vi "dfd_Interpret All Quantizers.vi"(11 "DFD_QSettings":T6[](array[typedef]) {"source" items=["Coef a/k"=0, "Coef b/v"=7, "Input"=1, "Output"=2, "Multiplicand"=3, "Product"=4, "Sum"=5, "Delay"=6, "Gain"=8]}) -> (3 "Fxp_QSettings":T1 {"source" items=["Coef a/k"=0, "Coef b/v"=7, "Input"=1, "Output"=2, "Multiplicand"=3, "Product"=4, "Sum"=5, "Delay"=6, "Gain"=8]})   [LabVIEW 2017, in "NI_DigFilterLicensed.lvlib"]
uses:
  <vilib>/addons/Digital Filter Design/NI_DigFilterLicensed.lvlib
  <vilib>/addons/Digital Filter Design/_Objects.llb/dfd_Internal Quantization Settings.ctl
  <vilib>/addons/Digital Filter Design/_Objects.llb/dfd_Internal Quantization Srcs.ctl
  <vilib>/addons/Digital Filter Design/SCLCodeGen.llb/Typedefs/dfd_SCL_Quantizers.ctl
  <vilib>/fxp/LVFixedPointRepBitsTypeDef.ctl
  <vilib>/fxp/LVFixedPointQuantizationPolicyTypeDef.ctl
  <vilib>/fxp/LVFixedPointOverflowPolicyTypeDef.ctl
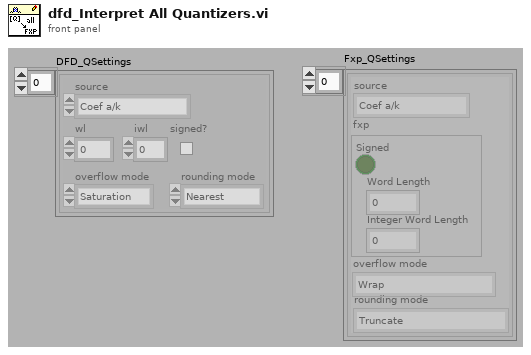
[diagram p1: front panel]
types:
  T1 = typedef "dfd_SCL_Quantizers.ctl" = cluster{"fxp":T2, "rounding mode":T3, "overflow mode":T4, "source":T5}[]
  T2 = typedef "LVFixedPointRepBitsTypeDef.ctl" = cluster{"Signed":bool, "Word Length":u32, "Integer Word Length":i32}
  T3 = typedef "LVFixedPointQuantizationPolicyTypeDef.ctl" = enum32{"Truncate", "Round-Half-Up (Asymmetric)", "Round-Half-Even"}
  T4 = typedef "LVFixedPointOverflowPolicyTypeDef.ctl" = enum32{"Wrap", "Saturate"}
  T5 = typedef "NI_DigFilterLicensed.lvlib/dfd_Internal Quantization Srcs.ctl" = u16
  T6 = typedef "NI_DigFilterLicensed.lvlib/dfd_Internal Quantization Settings.ctl" = cluster{"source":T5, "wl":i16, "iwl":i16, "overflow mode":enum16{"Saturation", "Wrap"}, "rounding mode":enum16{"Nearest", "Truncation"}, "signed?":bool}
  T7 = cluster{"fxp representation":T2, "rounding mode":T3, "overflow mode":T4, "source":T5}
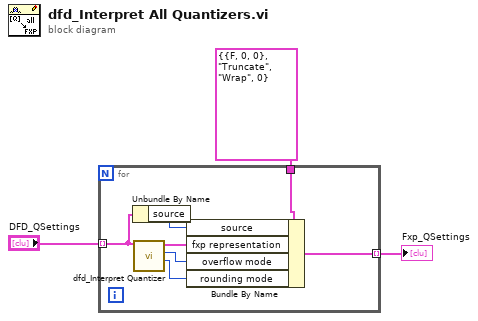
[diagram p0: block diagram]
diagram:
  n1 = for {
    tunnel: "DFD_QSettings" -> [w9] mode=indexing
    tunnel: T7 {"fxp representation"={"Signed"=FALSE, "Word Length"=0, "Integer Word Length"=0}, "rounding mode"=enum."Truncate", "overflow mode"=enum."Wrap", "source"=0} ("Cluster") -> [w10]
    tunnel: [w4] -> w1 mode=indexing
    n2 = Unbundle By Name(w9) -> ("source"=w8:T5)
    n3 = call <vilib>:"dfd_Interpret Quantizer.vi"("quantizer"=w9) -> ("rounding mode"=w5:T3, "overflow mode"=w6:T4, "fxp representation"=w7:T2)  [unwired: 8 out]
    n4 = Bundle By Name(cluster=w10, "source"=w8, "fxp representation"=w7, "overflow mode"=w6, "rounding mode"=w5) -> (w4:T7)
  }
  "Fxp_QSettings" <- w1
